vi "Test TCRS Update Ramp Rate While Running.vi"(8 "error in (no error)":errorcluster, 11 "Thermal Chamber Response Simlator Test In":refnum<class "Thermal Chamber Response Simlator Test.lvclass">) -> (0 "error out":errorcluster, 3 "Thermal Chamber Response Simlator Test Out":refnum<class "Thermal Chamber Response Simlator Test.lvclass">)   [LabVIEW 2020, in "Thermal Chamber Response Simlator Test.lvclass"]
uses:
  Thermal Chamber Response Simlator Test.lvclass
  C:/Program Files (x86)/National Instruments/LabVIEW 2020/vi.lib/Astemes/LUnit/Test Case.lvclass
  Thermal Chamber Response Simlator/Thermal Chamber Response Simlator.lvclass
  Thermal Chamber Response Simlator/Thermal Chamber Response Simlator.lvclass/Thermal Chamber Response Simlator.ctl
  <vilib>/Astemes/LUnit/Test Case.lvclass/Test Case.ctl
  <vilib>/Astemes/LUnit/Palette/Pass If Equal.vi/cbf50e99-f124-4847-863a-8e9794d3dede.vi
  <vilib>/Astemes/LUnit/Palette/Pass.vi
  <vilib>/Astemes/LUnit/Palette/Fail.vi
  <vilib>/Astemes/LUnit/Compare Variants.vi
  <vilib>/Astemes/LUnit/Describe Comparison.vi
  <vilib>/Astemes/LUnit/Set Assertion Type.vi
  <vilib>/Astemes/LUnit/Add test result.vi
  <vilib>/Astemes/LUnit/Variant to string.vi
  <vilib>/Astemes/LUnit/LUnit Record Assertion Result.vi
  <vilib>/Astemes/LUnit/LUnit Aggregate Assertion Results.vi
  <vilib>/Astemes/LUnit/Method Result/LUnit Merge Status.vi
  <vilib>/Astemes/LUnit/LUnit Concatenate result strings.vi
  Thermal Chamber Response Simlator/Private/Get Current Time if Not Set.vi
  <vilib>/Utility/Data Type/Get Type Information.vi
  <vilib>/Utility/LVClass/Get LV Class Name.vi
  <vilib>/Astemes/LUnit/Test Case.lvclass
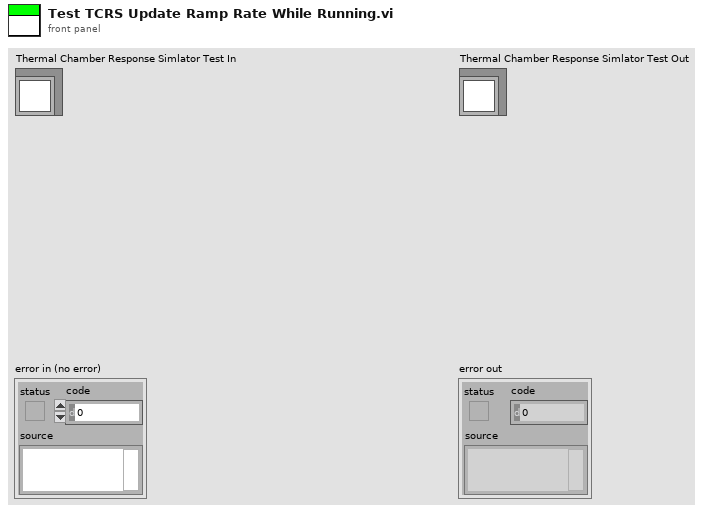
[diagram p1: front panel]
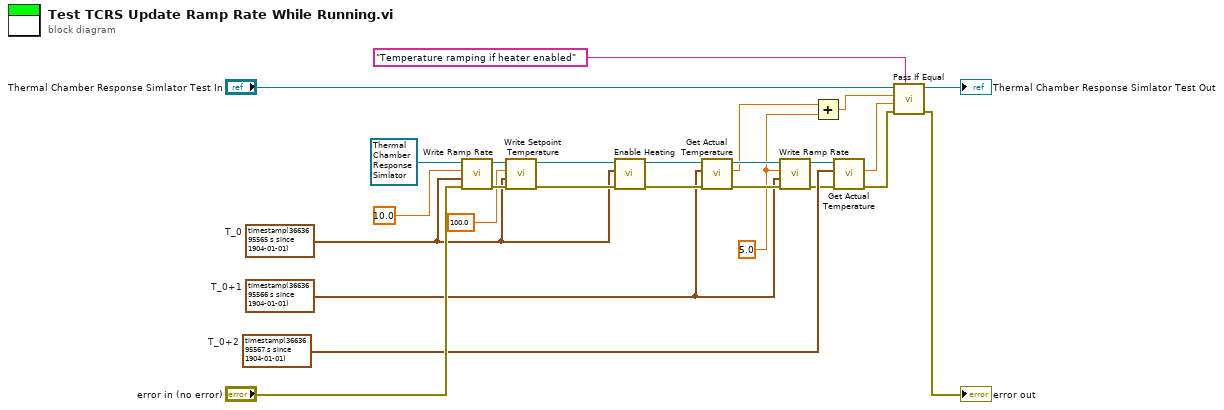
[diagram p0: block diagram]
diagram:
  w8 = timestamp(3663695567 s since 1904-01-01)  # T_0+2
  w2 = 5.0 ("Ramp Rate [degC/s]")
  w9 = timestamp(3663695566 s since 1904-01-01)  # T_0+1
  w11 = timestamp(3663695565 s since 1904-01-01)  # T_0
  n1 = call "Write Ramp Rate.vi"("error in (no error)"="error in (no error)", "Time Stamp"=w11, "Ramp Rate [degC/s]"=10.0, "Thermal Chamber Response Simlator In"=refnum<class "Thermal Chamber Response Simlator.lvclass"> refnum ("Thermal Chamber Response Simlator.lvclass")) -> ("error out"=w24:errorcluster, "Thermal Chamber Response Simlator Out"=w14:refnum<class "Thermal Chamber Response Simlator.lvclass">)  [unwired: 6 in]
  n2 = call "Write Setpoint Temperature.vi"("error in (no error)"=w24, "Update Time"=w11, "Setpoint Temperature [degC]"=100.0, "Thermal Chamber Response Simlator In"=w14) -> ("error out"=w15:errorcluster, "Thermal Chamber Response Simlator Out"=w13:refnum<class "Thermal Chamber Response Simlator.lvclass">)  [unwired: 6 in]
  n3 = call "Enable Heating.vi"("error in (no error)"=w15, "Start Time"=w11, "Thermal Chamber Response Simlator In"=w13) -> ("error out"=w18:errorcluster, "Thermal Chamber Response Simlator Out"=w17:refnum<class "Thermal Chamber Response Simlator.lvclass">)  [unwired: 7 in]
  n4 = call "Get Actual Temperature.vi"("error in (no error)"=w18, "Time Stamp"=w9, "Thermal Chamber Response Simlator In"=w17) -> ("error out"=w22:errorcluster, "Actual Temperature [degC]"=w3:dbl, "Thermal Chamber Response Simlator Out"=w10:refnum<class "Thermal Chamber Response Simlator.lvclass">)  [unwired: 6 in]
  n5 = call "Write Ramp Rate.vi"("error in (no error)"=w22, "Time Stamp"=w9, "Ramp Rate [degC/s]"=w2, "Thermal Chamber Response Simlator In"=w10) -> ("error out"=w6:errorcluster, "Thermal Chamber Response Simlator Out"=w7:refnum<class "Thermal Chamber Response Simlator.lvclass">)  [unwired: 6 in]
  n6 = Add(x=w3, y=w2) -> (x+y=w1:dbl)
  n7 = call "Get Actual Temperature.vi"("error in (no error)"=w6, "Time Stamp"=w8, "Thermal Chamber Response Simlator In"=w7) -> ("error out"=w5:errorcluster, "Actual Temperature [degC]"=w4:dbl)  [unwired: 6 in, 1 out]
  n8 = call <vilib>:"Pass If Equal.vi"("Description"="Temperature ramping if heater enabled", "error in (no error)"=w5, "Actual"=w4, "Expected"=w1, "LUnit Test Case In"="Thermal Chamber Response Simlator Test In") -> ("error out"=→"error out":errorcluster, "LUnit Test Case Out"=→"Thermal Chamber Response Simlator Test Out":refnum<class "Thermal Chamber Response Simlator Test.lvclass">)  [unwired: 5 in]
